vi "Get Value.vi"(8 "error in (no error)":errorcluster, 11 "String Item Configuration in":refnum<class "String Item Configuration.lvclass">) -> (0 "error out":errorcluster, 2 "Project Info Value":string, 3 "String Item Configuration out":refnum<class "String Item Configuration.lvclass">)   [LabVIEW 2013, in "Item Configuration.lvlib" / "String Item Configuration.lvclass"]
uses:
  String Item Configuration.lvclass
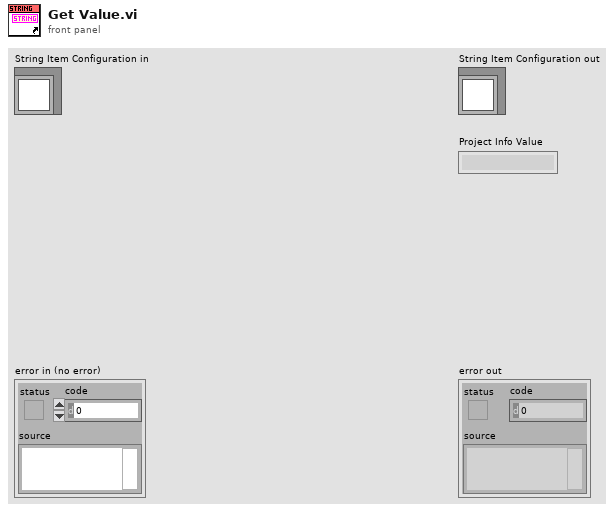
[diagram p1: front panel]
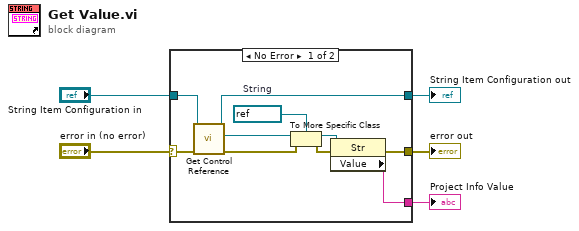
[diagram p0: block diagram]
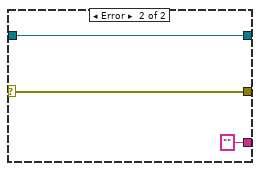
[diagram p2: hidden frame]
diagram:
  n1 = case shown="No Error" "error in (no error)" {
    selector: "error in (no error)" -> [w11 w18]
    tunnel: [w13 "" ("Value")] -> w5
    tunnel: [w12 w18] -> w4
    tunnel: "String Item Configuration in" -> [w10 w17]
    tunnel: [w9 w17] -> w1
    frame No Error {
      w14 = refnum<vi> refnum  # String
      n2 = call-dynamic "Get Control Reference.vi"("error in (no error)"=w11, "Item Configuration in"=w10) -> ("error out"=w8:errorcluster, "Control Reference"=w15:refnum<vi>, "Item Configuration out"=w9:refnum<class "String Item Configuration.lvclass">)  [unwired: 7 in]
      n3 = To More Specific Class(target class=w14, reference=w15, error in=w8) -> (specific class reference=w6:refnum<vi>, error out=w7:errorcluster)
      n4 = property class="Str"(reference=w6, error in=w7) -> (error out=w12:errorcluster, "Value"=w13:string)  [unwired: 1 out]
    }
    frame Error {
    }
  }
  "error out" <- w4
  "String Item Configuration out" <- w1
  "Project Info Value" <- w5
